vi "Teleop - Set Arm Position.vi"(11 "Switch Inputs":T1) -> ()   [LabVIEW 2015]
uses:
  Projects/FRC Operator Interface Control Board/controlBoard_LabVIEW/Switch_Input_TypeDef.ctl
  Robot Code/Arm Mode TypeDef.ctl
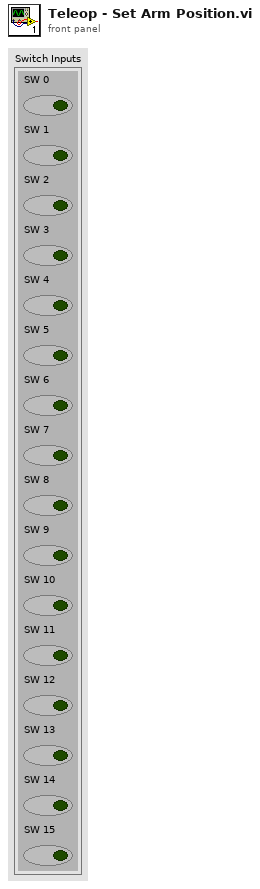
[diagram p1: front panel]
types:
  T1 = typedef "Switch_Input_TypeDef.ctl" = cluster{"SW 0":bool, "SW 1":bool, "SW 2":bool, "SW 3":bool, "SW 4":bool, "SW 5":bool, "SW 6":bool, "SW 7":bool, "SW 8":bool, "SW 9":bool, "SW 10":bool, "SW 11":bool, "SW 12":bool, "SW 13":bool, "SW 14":bool, "SW 15":bool}
  T2 = typedef "Arm Mode TypeDef.ctl" = enum16{"Disabled", "Locked", "Shoot Batter", "Shoot Close", "Shoot Far", "Human Player Load", "Low Bar / Goal", "Manual"}
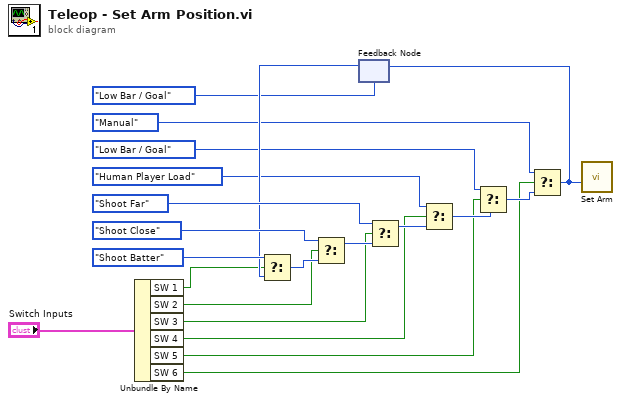
[diagram p0: block diagram]
diagram:
  n1 = Unbundle By Name("Switch Inputs") -> ("SW 1"=w8:bool, "SW 2"=w5:bool, "SW 3"=w6:bool, "SW 4"=w7:bool, "SW 5"=w12:bool, "SW 6"=w9:bool)
  n2 = feedback #1(Arm_Mode_TypeDef."Low Bar / Goal") -> (w17:T2)
  n3 = Select(t=Arm_Mode_TypeDef."Shoot Batter", s=w8, f=w17) -> (s? t:f=w16:T2)
  n4 = Select(t=Arm_Mode_TypeDef."Shoot Close", s=w5, f=w16) -> (s? t:f=w15:T2)
  n5 = Select(t=Arm_Mode_TypeDef."Shoot Far", s=w6, f=w15) -> (s? t:f=w14:T2)
  n6 = Select(t=Arm_Mode_TypeDef."Human Player Load", s=w7, f=w14) -> (s? t:f=w13:T2)
  n7 = Select(t=Arm_Mode_TypeDef."Low Bar / Goal", s=w12, f=w13) -> (s? t:f=w10:T2)
  n8 = Select(t=Arm_Mode_TypeDef."Manual", s=w9, f=w10) -> (s? t:f=w18:T2)
  n9 = feedback-in #1(w18) -> ()
  n10 = call "Set Arm.vi"("Arm Mode"=w18) -> ()  [unwired: 11 in]
